vi "PathPlanner_Trajectory_GetEndState.vi"(11 "PathPlannerTrajectory":T6 {"States"."HolonomicAngular\nvelocity Deg/Sec"."SIN" format="%13.4f"; "States"."HolonomicAngular\nvelocity Deg/Sec"."COS" format="%13.4f"; "States"."HolonomicAngular\nvelocity Deg/Sec"."VALUE" format="%13.4f"; "States"."HolonomicRotation"."SIN" format="%13.4f"; "States"."HolonomicRotation"."COS" format="%13.4f"; "States"."HolonomicRotation"."VALUE" format="%13.4f"; "States"."AngularVelocity"."SIN" format="%13.4f"; "States"."AngularVelocity"."COS" format="%13.4f"; "States"."AngularVelocity"."VALUE" format="%13.4f"; "States"."TrajectoryState"."POSE"."ROTATION"."SIN" format="%13.4f"; "States"."TrajectoryState"."POSE"."ROTATION"."COS" format="%13.4f"; "States"."TrajectoryState"."POSE"."ROTATION"."VALUE" format="%13.4f"; "States"."TrajectoryState"."POSE"."TRANSLATION"."Y" format="%14.3f"; "States"."TrajectoryState"."POSE"."TRANSLATION"."X" format="%14.3f"; "States"."AngularAcceleration"."SIN" format="%13.4f"; "States"."AngularAcceleration"."COS" format="%13.4f"; "States"."AngularAcceleration"."VALUE" format="%13.4f"}) -> (3 "PathPlannerState":T1={"AngularAcceleration"={"VALUE"=0.0, "COS"=1.0, "SIN"=0.0}, "PositionMeters"=0.0, "TrajectoryState"={"TimeSeconds"=0.0, "Velocity"=0.0, "Acceleration"=0.0, "POSE"={"TRANSLATION"={"X"=0.0, "Y"=0.0}, "ROTATION"={"VALUE"=0.0, "COS"=1.0, "SIN"=0.0}}, "Curvature"=0.0}, "AngularVelocity"={"VALUE"=0.0, "COS"=1.0, "SIN"=0.0}, "HolonomicRotation"={"VALUE"=0.0, "COS"=1.0, "SIN"=0.0}, "CurveRadius"=0.0, "DeltaPos"=0.0, "HolonomicAngular\nvelocity Deg/Sec"={"VALUE"=0.0, "COS"=1.0, "SIN"=0.0}} {"HolonomicAngular\nvelocity Deg/Sec"."SIN" format="%13.4f"; "HolonomicAngular\nvelocity Deg/Sec"."COS" format="%13.4f"; "HolonomicAngular\nvelocity Deg/Sec"."VALUE" format="%13.4f"; "HolonomicRotation"."SIN" format="%13.4f"; "HolonomicRotation"."COS" format="%13.4f"; "HolonomicRotation"."VALUE" format="%13.4f"; "AngularVelocity"."SIN" format="%13.4f"; "AngularVelocity"."COS" format="%13.4f"; "AngularVelocity"."VALUE" format="%13.4f"; "TrajectoryState"."POSE"."ROTATION"."SIN" format="%13.4f"; "TrajectoryState"."POSE"."ROTATION"."COS" format="%13.4f"; "TrajectoryState"."POSE"."ROTATION"."VALUE" format="%13.4f"; "TrajectoryState"."POSE"."TRANSLATION"."Y" format="%14.3f"; "TrajectoryState"."POSE"."TRANSLATION"."X" format="%14.3f"; "AngularAcceleration"."SIN" format="%13.4f"; "AngularAcceleration"."COS" format="%13.4f"; "AngularAcceleration"."VALUE" format="%13.4f"})   [LabVIEW 2019, in "PathPlanner.lvlib"]
doc: "Get the end state of the path\n\nInputs:\n -- PathPlannerTraectory -- PathPlanner Trajectory data cluster\n\nOutputs:\n - PathPlannerState -- The last state in the path"
uses:
  PathPlannerTrajectory.ctl
  PathPlannerState.ctl
  <vilib>/Rock Robotics/WPI/ThirdParty/JAS_Junk/TrajLib/TypeDef/ROTATION2D.ctl
  <vilib>/Rock Robotics/WPI/ThirdParty/JAS_Junk/TrajLib/TypeDef/TRAJ_STATE.ctl
  <vilib>/Rock Robotics/WPI/ThirdParty/JAS_Junk/TrajLib/TypeDef/POSE2D.ctl
  <vilib>/Rock Robotics/WPI/ThirdParty/JAS_Junk/TrajLib/TypeDef/TRANSLATION2D.ctl
  PathPlanner.lvlib
  <vilib>/Rock Robotics/WPI/ThirdParty/JAS_Junk/TrajLib/Trajectory_Library.lvlib
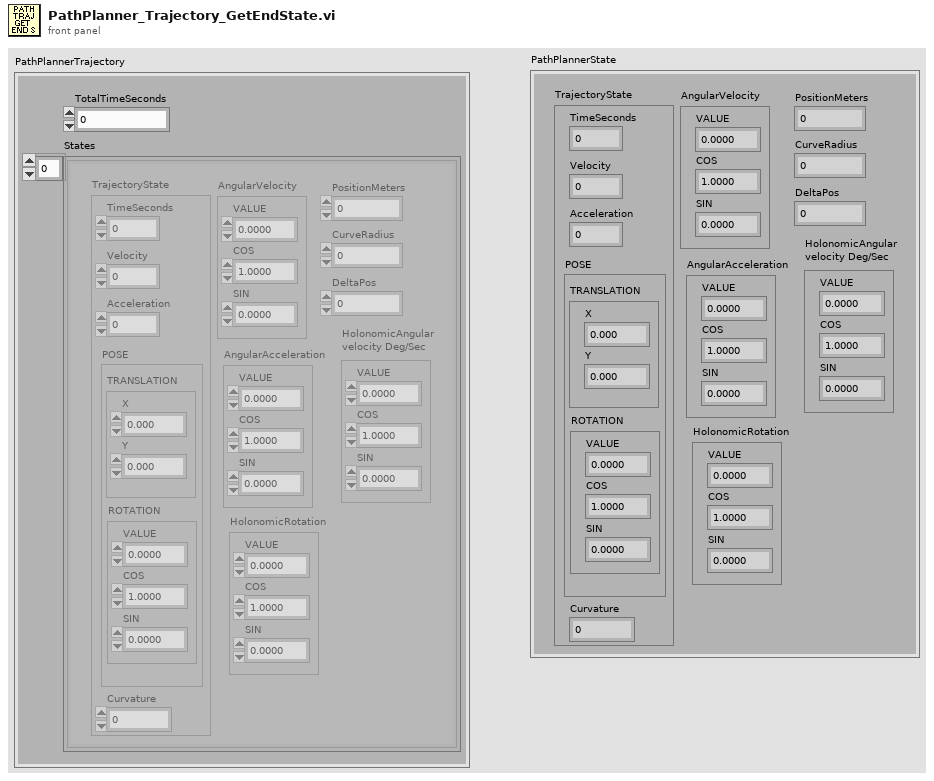
[diagram p1: front panel]
types:
  T1 = typedef "PathPlanner.lvlib/PathPlannerState.ctl" = cluster{"AngularAcceleration":T2, "PositionMeters":dbl, "TrajectoryState":T3, "AngularVelocity":T2, "HolonomicRotation":T2, "CurveRadius":dbl, "DeltaPos":dbl, "HolonomicAngular\nvelocity Deg/Sec":T2}
  T2 = typedef "Trajectory_Library.lvlib/ROTATION2D.ctl" = cluster{"VALUE":dbl, "COS":dbl, "SIN":dbl}
  T3 = typedef "Trajectory_Library.lvlib/TRAJ_STATE.ctl" = cluster{"TimeSeconds":dbl, "Velocity":dbl, "Acceleration":dbl, "POSE":T4, "Curvature":dbl}
  T4 = typedef "Trajectory_Library.lvlib/POSE2D.ctl" = cluster{"TRANSLATION":T5, "ROTATION":T2}
  T5 = typedef "Trajectory_Library.lvlib/TRANSLATION2D.ctl" = cluster{"X":dbl, "Y":dbl}
  T6 = typedef "PathPlanner.lvlib/PathPlannerTrajectory.ctl" = cluster{"TotalTimeSeconds":dbl, "States":T1[]}
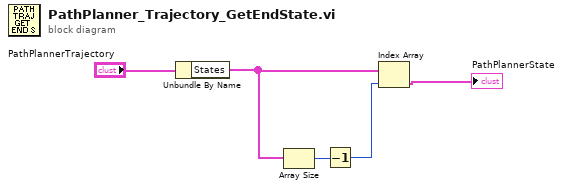
[diagram p0: block diagram]
diagram:
  n1 = Unbundle By Name("PathPlannerTrajectory") -> ("States"=w4:T1[])
  n2 = Array Size(array=w4) -> (size(s)=w3:i32)
  n3 = Decrement(x=w3) -> (x-1=w2:i32)
  n4 = Index Array(array=w4, index=w2) -> (element=→"PathPlannerState":T1)
